vi "Auto Play Path.vi"(8 "Operation":T3, 9 "Auto Data":T2, 10 "Motors":T4={"Drive Motors (NEO)"={"Left Front"={"DeviceStatus"={"status"=FALSE, "code"=0, "source"=""}, "Type"=enum."PWM", "PWM"={"PWM Channel"=enum."PWM 0", "DeadBand"={"Name"="", "maxPositivePwm"=0, "minPositivePwm"=0, "centerPwm"=0, "maxNegativePwm"=0, "minNegativePwm"=0, "angularRange"=0}}, "CAN"={"Device Number"=0, "SetOutput VI Ref"=variant, "GetOutput VI Ref"=variant, "Enable VI Ref"=variant, "Disable VI Ref"=variant, "Data"=variant}, "Invert"=FALSE, "DIO PWM"={"PWM \"Enable\" Channel"=enum."PWM 0", "DIOChannel"=enum."DIO 0", "PWM Rate"=0.0}}, "Left Back"={"DeviceStatus"={"status"=FALSE, "code"=0, "source"=""}, "Type"=enum."PWM", "PWM"={"PWM Channel"=enum."PWM 0", "DeadBand"={"Name"="", "maxPositivePwm"=0, "minPositivePwm"=0, "centerPwm"=0, "maxNegativePwm"=0, "minNegativePwm"=0, "angularRange"=0}}, "CAN"={"Device Number"=0, "SetOutput VI Ref"=variant, "GetOutput VI Ref"=variant, "Enable VI Ref"=variant, "Disable VI Ref"=variant, "Data"=variant}, "Invert"=FALSE, "DIO PWM"={"PWM \"Enable\" Channel"=enum."PWM 0", "DIOChannel"=enum."DIO 0", "PWM Rate"=0.0}}, "Right Front"={"DeviceStatus"={"status"=FALSE, "code"=0, "source"=""}, "Type"=enum."PWM", "PWM"={"PWM Channel"=enum."PWM 0", "DeadBand"={"Name"="", "maxPositivePwm"=0, "minPositivePwm"=0, "centerPwm"=0, "maxNegativePwm"=0, "minNegativePwm"=0, "angularRange"=0}}, "CAN"={"Device Number"=0, "SetOutput VI Ref"=variant, "GetOutput VI Ref"=variant, "Enable VI Ref"=variant, "Disable VI Ref"=variant, "Data"=variant}, "Invert"=FALSE, "DIO PWM"={"PWM \"Enable\" Channel"=enum."PWM 0", "DIOChannel"=enum."DIO 0", "PWM Rate"=0.0}}, "Right Back"={"DeviceStatus"={"status"=FALSE, "code"=0, "source"=""}, "Type"=enum."PWM", "PWM"={"PWM Channel"=enum."PWM 0", "DeadBand"={"Name"="", "maxPositivePwm"=0, "minPositivePwm"=0, "centerPwm"=0, "maxNegativePwm"=0, "minNegativePwm"=0, "angularRange"=0}}, "CAN"={"Device Number"=0, "SetOutput VI Ref"=variant, "GetOutput VI Ref"=variant, "Enable VI Ref"=variant, "Disable VI Ref"=variant, "Data"=variant}, "Invert"=FALSE, "DIO PWM"={"PWM \"Enable\" Channel"=enum."PWM 0", "DIOChannel"=enum."DIO 0", "PWM Rate"=0.0}}}, "Steer Motors (NEO)"={"Left Front"={"DeviceStatus"={"status"=FALSE, "code"=0, "source"=""}, "Type"=enum."PWM", "PWM"={"PWM Channel"=enum."PWM 0", "DeadBand"={"Name"="", "maxPositivePwm"=0, "minPositivePwm"=0, "centerPwm"=0, "maxNegativePwm"=0, "minNegativePwm"=0, "angularRange"=0}}, "CAN"={"Device Number"=0, "SetOutput VI Ref"=variant, "GetOutput VI Ref"=variant, "Enable VI Ref"=variant, "Disable VI Ref"=variant, "Data"=variant}, "Invert"=FALSE, "DIO PWM"={"PWM \"Enable\" Channel"=enum."PWM 0", "DIOChannel"=enum."DIO 0", "PWM Rate"=0.0}}, "Left Back"={"DeviceStatus"={"status"=FALSE, "code"=0, "source"=""}, "Type"=enum."PWM", "PWM"={"PWM Channel"=enum."PWM 0", "DeadBand"={"Name"="", "maxPositivePwm"=0, "minPositivePwm"=0, "centerPwm"=0, "maxNegativePwm"=0, "minNegativePwm"=0, "angularRange"=0}}, "CAN"={"Device Number"=0, "SetOutput VI Ref"=variant, "GetOutput VI Ref"=variant, "Enable VI Ref"=variant, "Disable VI Ref"=variant, "Data"=variant}, "Invert"=FALSE, "DIO PWM"={"PWM \"Enable\" Channel"=enum."PWM 0", "DIOChannel"=enum."DIO 0", "PWM Rate"=0.0}}, "Right Front"={"DeviceStatus"={"status"=FALSE, "code"=0, "source"=""}, "Type"=enum."PWM", "PWM"={"PWM Channel"=enum."PWM 0", "DeadBand"={"Name"="", "maxPositivePwm"=0, "minPositivePwm"=0, "centerPwm"=0, "maxNegativePwm"=0, "minNegativePwm"=0, "angularRange"=0}}, "CAN"={"Device Number"=0, "SetOutput VI Ref"=variant, "GetOutput VI Ref"=variant, "Enable VI Ref"=variant, "Disable VI Ref"=variant, "Data"=variant}, "Invert"=FALSE, "DIO PWM"={"PWM \"Enable\" Channel"=enum."PWM 0", "DIOChannel"=enum."DIO 0", "PWM Rate"=0.0}}, "Right Back"={"DeviceStatus"={"status"=FALSE, "code"=0, "source"=""}, "Type"=enum."PWM", "PWM"={"PWM Channel"=enum."PWM 0", "DeadBand"={"Name"="", "maxPositivePwm"=0, "minPositivePwm"=0, "centerPwm"=0, "maxNegativePwm"=0, "minNegativePwm"=0, "angularRange"=0}}, "CAN"={"Device Number"=0, "SetOutput VI Ref"=variant, "GetOutput VI Ref"=variant, "Enable VI Ref"=variant, "Disable VI Ref"=variant, "Data"=variant}, "Invert"=FALSE, "DIO PWM"={"PWM \"Enable\" Channel"=enum."PWM 0", "DIOChannel"=enum."DIO 0", "PWM Rate"=0.0}}}, "PigeonIMUDevRef"={"DeviceStatus"={"status"=FALSE, "code"=0, "source"=""}, "Device Number"=0, "Type"=352321536, "Device ID"=0, "Handle"=0, "UsageFrame"=0, "Library Path"=path ""}, "Radii (ft)"={"Left Front Position"=[], "Left Back Position"=[], "Right Front Position"=[], "Right Back Position"=[]}} {"Radii (ft)"."Right Back Position" format="%.2f"; "Radii (ft)"."Right Front Position" format="%.2f"; "Radii (ft)"."Left Back Position" format="%.2f"; "Radii (ft)"."Left Front Position" format="%.2f"; "PigeonIMUDevRef"."Type" items=["CAN"=352321536, "TalonSRX"=33554432]}, 11 "Is Red Alliance":bool) -> (0 "Auto Done?":bool)   [LabVIEW 2025]
uses:
  swerve-template/Type Definitions/Hardware/Swerve Drives/(NEO-NEO-ThroughBore-Pigeon2) Swerve.ctl
  swerve-template/Type Definitions/Hardware/4 Motor Sets/(NEO & NEO 550) 4 Motor Set.ctl
  <vilib>/Rock Robotics/WPI/MotorControl/WPI_MotorControlDeviceRef.ctl
  <vilib>/Rock Robotics/WPI/MotorControl/WPI_MotorControlType.ctl
  <vilib>/Rock Robotics/SystemInterfaces/DIO/FPGA_DIOPWMChannel.ctl
  <vilib>/Rock Robotics/WPI/PWM/WPI_PWMDeadband.ctl
  <vilib>/Rock Robotics/SystemInterfaces/DIO/FPGA_DIOChannel.ctl
  <vilib>/Rock Robotics/WPI/ThirdParty/Phoenix-LabVIEW/Pigeon IMU/CTRE_PigeonIMU_DeviceRef.ctl
  <vilib>/Rock Robotics/WPI/ThirdParty/Phoenix-LabVIEW/Pigeon IMU/CTRE_PigeonIMU_ConnectionType.ctl
  swerve-template/Type Definitions/Data/Pod Positions.ctl
  Implementation/Drive Operations.ctl
  swerve-template/Type Definitions/Data/Robot Velocities.ctl
  <vilib>/Rock Robotics/WPI/ThirdParty/REV Robotics/REVLib/Typedef/Spark MAX Control Type.ctl
  <vilib>/Platform/TimedLoop/XDataNode/timing_clust.ctl
  <vilib>/Platform/TimedLoop/XDataNode/nitl_modes.ctl
  <vilib>/Platform/TimedLoop/XDataNode/wakeup.ctl
  <vilib>/Rock Robotics/WPI/DriverStation/WPI_DriverStationRobotMode2.ctl
  Framework/Robot Global Data.vi
  <vilib>/Platform/TimedLoop/XDataNode/XDataNode.xnode
  <vilib>/Platform/TimedLoop/XDataNode/XDNodeRunTimeDep.lvlib
panel:
  out "dt array":dbl[](array[numeric])
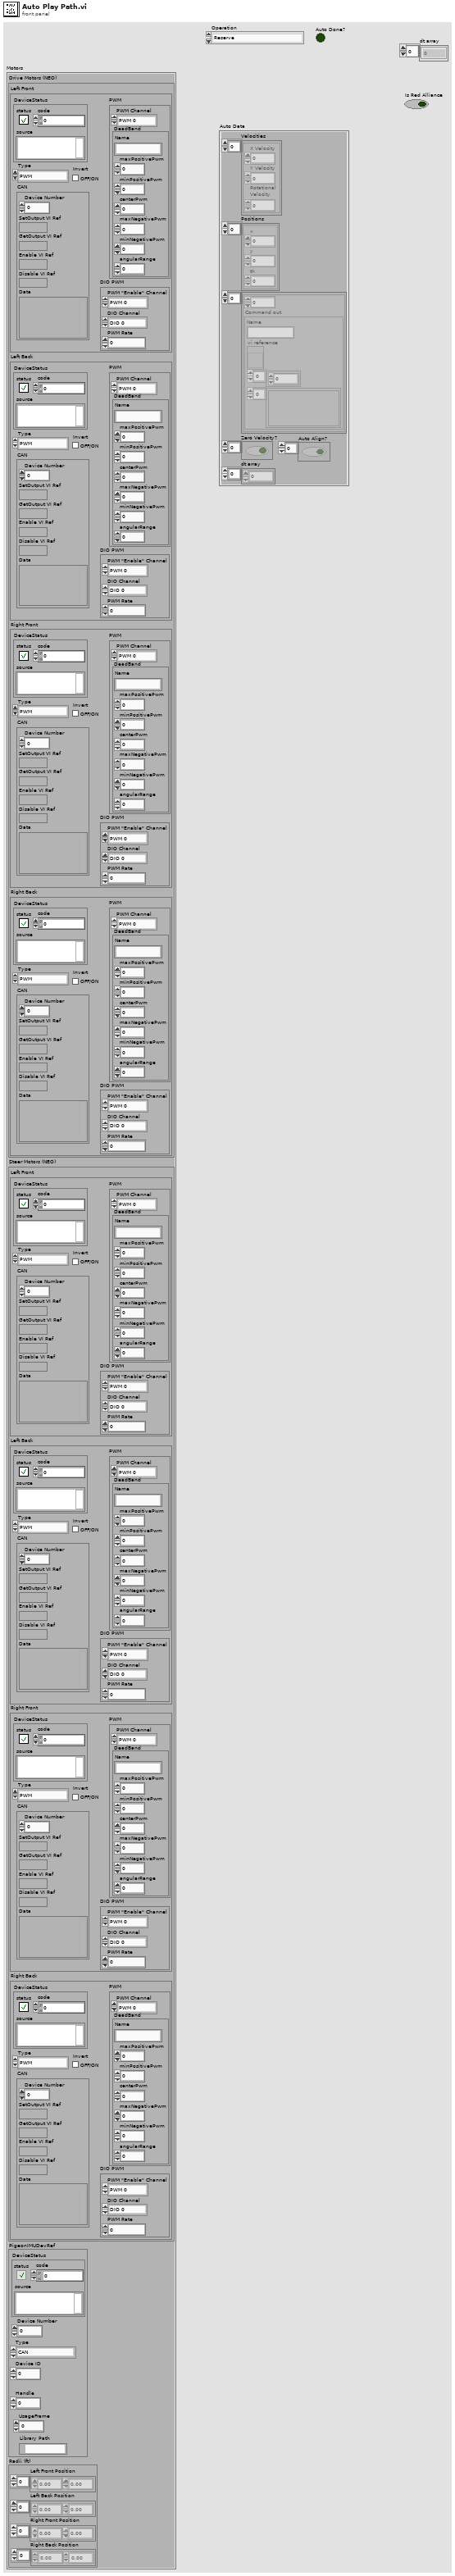
[diagram p1: front panel]
types:
  T1 = typedef "Robot Velocities.ctl" = cluster{"X Velocity":dbl, "Y Velocity":dbl, "Rotational \nVelocity":dbl}
  T2 = cluster{"Velocities":T1[], "Positions":cluster{"x":dbl, "y":dbl, "th":dbl}[], cluster{dbl, "Command out":cluster{"Name":string, "vi reference":refnum<vi>, i32[], variant[]}}[], "Zero Velocity?":bool[], "dt array":dbl[], "Auto Align?":bool[]}
  T3 = typedef "Drive Operations.ctl" = enum16{"Reserve", "Read Current", "Immediate", "Calibrate", "Auto", "Set Center of Rotation", "Point to Hub"}
  T4 = typedef "(NEO-NEO-ThroughBore-Pigeon2) Swerve.ctl" = cluster{"Drive Motors (NEO)":T5, "Steer Motors (NEO)":T5, "PigeonIMUDevRef":T11, "Radii (ft)":T13}
  T5 = typedef "(NEO & NEO 550) 4 Motor Set.ctl" = cluster{"Left Front":T6, "Left Back":T6, "Right Front":T6, "Right Back":T6}
  T6 = typedef "WPI_MotorControlDeviceRef.ctl" = cluster{"DeviceStatus":errorcluster, "Type":T7, "PWM":cluster{"PWM Channel":T8, "DeadBand":T9}, "CAN":cluster{"Device Number":u8, "SetOutput VI Ref":variant, "GetOutput VI Ref":variant, "Enable VI Ref":variant, "Disable VI Ref":variant, "Data":variant}, "Invert":bool, "DIO PWM":cluster{"PWM \"Enable\" Channel":T8, "DIOChannel":T10, "PWM Rate":dbl}}
  T7 = typedef "WPI_MotorControlType.ctl" = enum16{"PWM", "CAN", "DIO PWM"}
  T8 = typedef "FPGA_DIOPWMChannel.ctl" = enum8{"PWM 0", "PWM 1", "PWM 2", "PWM 3", "PWM 4", "PWM 5", "PWM 6", "PWM 7", "PWM 8", "PWM 9", "PWM MXP 0", "PWM MXP 1", "PWM MXP 2", "PWM MXP 3", "PWM MXP 4", "PWM MXP 5", "PWM MXP 6", "PWM MXP 7", "PWM MXP 8", "PWM MXP 9", "Invalid"}
  T9 = typedef "WPI_PWMDeadband.ctl" = cluster{"Name":string, "maxPositivePwm":i32, "minPositivePwm":i32, "centerPwm":i32, "maxNegativePwm":i32, "minNegativePwm":i32, "angularRange":u16}
  T10 = typedef "FPGA_DIOChannel.ctl" = enum8{"DIO 0", "DIO 1", "DIO 2", "DIO 3", "DIO 4", "DIO 5", "DIO 6", "DIO 7", "DIO 8", "DIO 9", "DIO MXP 0", "DIO MXP 1", "DIO MXP 2", "DIO MXP 3", "DIO MXP 4", "DIO MXP 5", "DIO MXP 6", "DIO MXP 7", "DIO MXP 8", "DIO MXP 9", "DIO MXP 10", "DIO MXP 11", "DIO MXP 12", "DIO MXP 13", "DIO MXP 14", "DIO MXP 15", "SPI Port CS1", "SPI Port CS2", "SPI Port CS3", "SPI Port MISO", "SPI Port MOSI", "Invalid"}
  T11 = typedef "CTRE_PigeonIMU_DeviceRef.ctl" = cluster{"DeviceStatus":errorcluster, "Device Number":u8, "Type":T12, "Device ID":u32, "Handle":u64, "UsageFrame":u32, "Library Path":path}
  T12 = typedef "CTRE_PigeonIMU_ConnectionType.ctl" = u32
  T13 = typedef "Pod Positions.ctl" = cluster{"Left Front Position":dbl[], "Left Back Position":dbl[], "Right Front Position":dbl[], "Right Back Position":dbl[]}
  T14 = cluster{"Time (s)":dbl, "Command out":cluster{"Name":string, "vi reference":refnum<vi>, i32[], variant[]}}
  T15 = typedef "Spark MAX Control Type.ctl" = enum16{"Percent VBus", "Voltage", "Velocity", "Position", "Smart Motion", "Current", "Smart Velocity", "MAXMotion Position", "MAXMotion Velocity"}
  T16 = cluster{"Left Front":dbl, "Left Back":dbl, "Right Front":dbl, "Right Back":dbl}
  T17 = cluster{dbl, "Command out":cluster{"Name":string, "vi reference":refnum<vi>, i32[], variant[]}}[]
  T18 = typedef "XDNodeRunTimeDep.lvlib/timing_clust.ctl" = cluster{"Expected End [f-1]":u64, "Actual End [f-1]":u64, "Finished Late? [f-1]":bool, "Expected End [i-1]":u64, "Actual End [i-1]":u64, "Finished Late? [i-1]":bool, "Expected Start [i]":u64, "Actual Start [i]":u64, "Expected Start [f]":u64, "Actual Start [f]":u64, "Source Name":string, "Structure Name":string, "Period":i64, "Deadline":i64, "Offset":i64, "Start":i64, "Priority":i32, "Timeout":i32, "Mode":T19, "Wakeup Reason":T20, "Error":errorcluster, "Source Type":string, "Secondary Source Type":string, "Global End Time":u64, "Global Start Time":u64, "Frame Duration":u64, "Iteration Duration":u64, "Assigned CPU":i32, "I/O Scan Engine Mode":u32}
  T19 = typedef "XDNodeRunTimeDep.lvlib/nitl_modes.ctl" = enum32{"No Change", "Process missed periods, maintain original phase", "Discard missed periods, maintain original phase", "Process missed periods, ignore original phase", "Discard missed periods, ignore original phase"}
  T20 = typedef "XDNodeRunTimeDep.lvlib/wakeup.ctl" = enum32{"Normal", "Aborted", "Asynchronous wakeup", "Timing source error", "Timed loop error", "Timeout"}
  T21 = typedef "WPI_DriverStationRobotMode2.ctl" = enum16{"Autonomous Disabled", "Autonomous Enabled", "Teleop Disabled", "Teleop Enabled", "Disconnected", "Finish", "Test Disabled", "Test Enabled", "Emergency Stopped"}
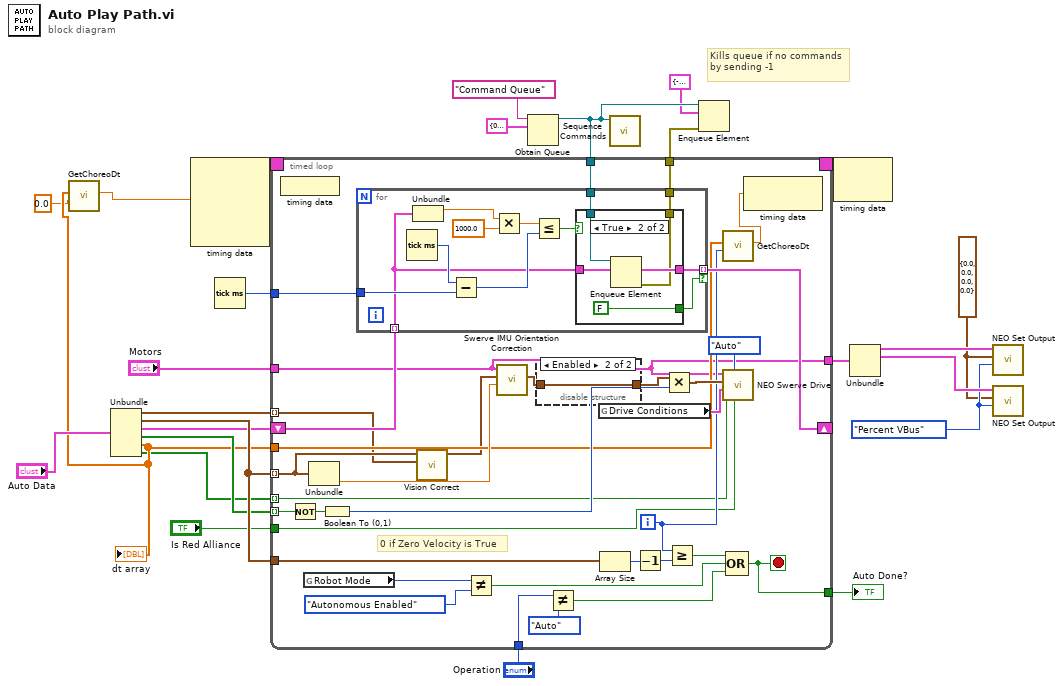
[diagram p0: block diagram]
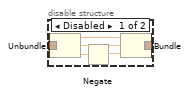
[diagram p2: hidden frame]
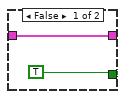
[diagram p3: hidden frame]
diagram:
  w15 = Spark_MAX_Control_Type."Percent VBus" ("Control Mode")
  w14 = T16 {"Left Front"=0.0, "Left Back"=0.0, "Right Front"=0.0, "Right Back"=0.0} ("Setpoints")
  # "Kills queue if no commands by sending -1"
  n1 = Unbundle("Auto Data") -> ("Velocities"=w21:T1[], "Positions"=w22:cluster{"x":dbl, "y":dbl, "th":dbl}[], w1:T17, "Zero Velocity?"=w8:bool[], "dt array"=w6:dbl[], "Auto Align?"=w3:bool[])
  "dt array" <- w6
  n2 = call "GetChoreoDt.vi"("index"=0.0, "dt array"=w6) -> ("dt"=w5:dbl)  [unwired: 8 in, 1 out]
  n3 = node-c288(w5) -> (w26:T18)  [unwired: 3 in]
  n4 = Tick Count (ms)() -> (millisecond timer value=w23:u32)
  n5 = Obtain Queue(name (unnamed)="Command Queue", element data type=T14 {"Time (s)"=0.0, "Command out"={"Name"="", "vi reference"=refnum, [], []}} ("element")) -> (queue out=w11:refnum<queue>)  [unwired: 3 in, 2 out]
  n6 = timed-loop {
    timing: w26 -> [_]
    timing-out: [_] -> w25
    tunnel: "Motors" -> [w34]
    tunnel: [w34] -> w13
    tunnel: w21 -> [w29] mode=indexing
    tunnel: w22 -> [w30] mode=indexing
    tunnel: w22 -> [w60]
    tunnel: w23 -> [w59]
    tunnel: w11 -> [w57]
    shift-right: [w55] -> _
    shift-left: w1 -> [w54]
    tunnel: w8 -> [w44] mode=indexing
    tunnel: [w47] -> w24
    tunnel: "Operation" -> [w43]
    tunnel: [w42] -> w10
    tunnel: w6 -> [w37]
    tunnel: w3 -> [w31] mode=indexing
    tunnel: "Is Red Alliance" -> [w27]
    i -> [w36]
    stop <- w47 stop-if-true
    # "0 if Zero Velocity is True"
    n7 = node-c288() -> ()  [unwired: 1 in]
    n8 = Not(x=w44) -> (.not. x?=w51:bool)
    n9 = global read "Robot Global Data.vi" "Robot Mode"() -> (w53:T21)
    n10 = Unbundle(w30) -> ("th"=w40:dbl)  [unwired: 2 out]
    n11 = Boolean To (0,1)(Boolean=w51) -> (0, 1=w50:i16)
    n12 = for {
      tunnel: w59 -> [w78]
      tunnel: w57 -> [w72]
      tunnel: w54 -> [w69] mode=indexing
      tunnel: [w71] -> w55 mode=indexing if=w70
      tunnel: [w68] -> w42
      n13 = Tick Count (ms)() -> (millisecond timer value=w79:u32)
      n14 = Unbundle(w69) -> (w77:dbl)  [unwired: 1 out]
      n15 = Subtract(x=w79, y=w78) -> (x-y=w74:u32)
      n16 = Multiply(x=w77, y=1000.0) -> (x*y=w75:dbl)
      n17 = Less Or Equal?(x=w75, y=w74) -> (x <= y?=w73:bool)
      n18 = case shown="True" w73 {
        tunnel: w72 -> [_ w85]
        tunnel: w69 -> [w80 w84]
        tunnel: [w80 w84] -> w71
        tunnel: [TRUE FALSE] -> w70
        tunnel: [_ w82] -> w68
        frame False {
        }
        frame True {
          n19 = Enqueue Element(queue=w85, element=w84) -> (error out=w82:errorcluster)  [unwired: 2 in, 2 out]
        }
      }
    }
    n20 = call "Vision Correct.vi"("Robot Velocities In"=w29, "Robot Position Setpoint"=w30) -> ("Robot Velocities Out"=w28:T1)  [unwired: 9 in]
    n21 = Not Equal?(x=w53, y=WPI_DriverStationRobotMode2."Autonomous Enabled") -> (x != y?=w48:bool)
    n22 = call "Swerve IMU Orientation Correction.vi"("Setpoint"=w40, "Robot Velocities In"=w28, "Motors In"=w34) -> ("Robot Velocities Out"=w33:T1)  [unwired: 7 in, 1 out]
    n23 = disable-structure shown="Enabled" {
      disable-tunnel: w33 -> [w66 w67]
      disable-tunnel: [w61 w67] -> w32
      frame Disabled {
        n24 = Unbundle(w66) -> ("X Velocity"=w62:dbl, "Y Velocity"=w63:dbl, "Rotational \nVelocity"=w65:dbl)
        n25 = Negate(x=w65) -> (-x=w64:dbl)
        n26 = Bundle("X Velocity"=w62, "Y Velocity"=w63, w64) -> (w61:cluster{"X Velocity":dbl, "Y Velocity":dbl, dbl})  [unwired: 1 in]
      }
      frame Enabled {
      }
    }
    n27 = Not Equal?(x=w43, y=Drive_Operations."Auto") -> (x != y?=w46:bool)
    n28 = global read "Robot Global Data.vi" "Drive Conditions"() -> (w41:cluster{"Field Centric":bool})
    n29 = Array Size(array=w60) -> (size(s)=w38:i32)
    n30 = Decrement(x=w38) -> (x-1=w39:i32)
    n31 = Multiply(x=w32, y=w50) -> (x*y=w49:T1)
    n32 = Greater Or Equal?(x=w36, y=w39) -> (x >= y?=w58:bool)
    n33 = call "GetChoreoDt.vi"("index"=w36, "dt array"=w37) -> ("dt"=w35:dbl)  [unwired: 8 in, 1 out]
    n34 = call "NEO Swerve Drive.vi"("Is Red Alliance"=w27, "Operation"=Drive_Operations."Auto", "Auto Align?"=w31, "Drive Conditions"=w41, "Robot Velocities"=w49, "Swerve Drive"=w34) -> ()  [unwired: 5 in, 1 out]
    n35 = Compound Arithmetic op=OR(w58, w48, w46) -> (w47:bool)
    n36 = node-c288(w35) -> ()  [unwired: 1 out]
  }
  "Auto Done?" <- w24
  n37 = call "Sequence Commands.vi"("queue in"=w11) -> ()  [unwired: 11 in]
  n38 = Enqueue Element(queue=w11, element=T14 {"Time (s)"=-1.0, "Command out"={"Name"="", "vi reference"=refnum, [], []}}, error in (no error)=w10) -> ()  [unwired: 1 in, 3 out]
  n39 = node-c288(w25) -> ()  [unwired: 1 out]
  n40 = Unbundle(w13) -> ("Drive Motors (NEO)"=w17:T5, "Steer Motors (NEO)"=w16:T5)  [unwired: 2 out]
  n41 = call "NEO Set Output.vi"("Control Mode"=w15, "Setpoints"=w14, "Motors"=w17) -> ()  [unwired: 9 in]
  n42 = call "NEO Set Output.vi"("Control Mode"=w15, "Setpoints"=w14, "Motors"=w16) -> ()  [unwired: 9 in]
